vi "SRV_Shutdown Flag.vi"(7 "Shutdown Flag":bool, 11 "error in (no error)":errorcluster, 12 "Method (Get)":enum16{"Get", "Set"}(ring)) -> (8 "Shutdown Flag out":bool, 15 "error out":errorcluster)   [LabVIEW 2009]
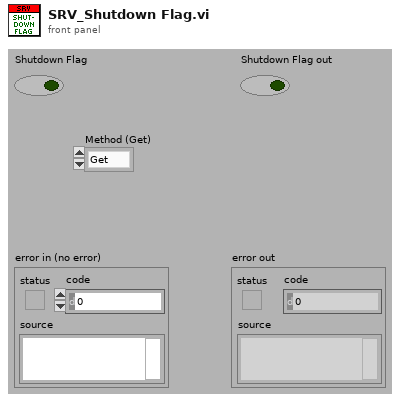
[diagram p1: front panel]
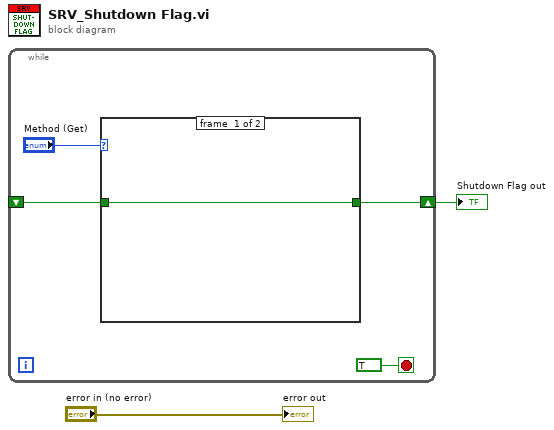
[diagram p0: block diagram]
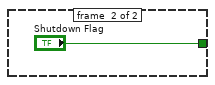
[diagram p2: hidden frame]
diagram:
  n1 = while {
    shift-right: [w3] -> w2
    shift-left: _ -> [w5]
    stop <- TRUE stop-if-true
    n2 = case shown="\"Set\"" "Method (Get)" {
      tunnel: w5 -> [w7 _]
      tunnel: [w7 "Shutdown Flag"] -> w3
      frame #0 {
      }
      frame #1 {
      }
    }
  }
  "Shutdown Flag out" <- w2
  "error out" <- "error in (no error)"
